vi "mediaBalls_v2.vi"(10 "Lado":enum16{"Esquerdo", "Direito"}(ring) caption="Enum", 11 "Array Ball Pose + CamID":T1(array[cluster])) -> (3 "Ball out":cluster{"x":dbl, "y":dbl})   [LabVIEW 2018]
panel:
  in  "cluster":cluster{"x":dbl, "y":dbl}
  in  "Field Size 2":T2
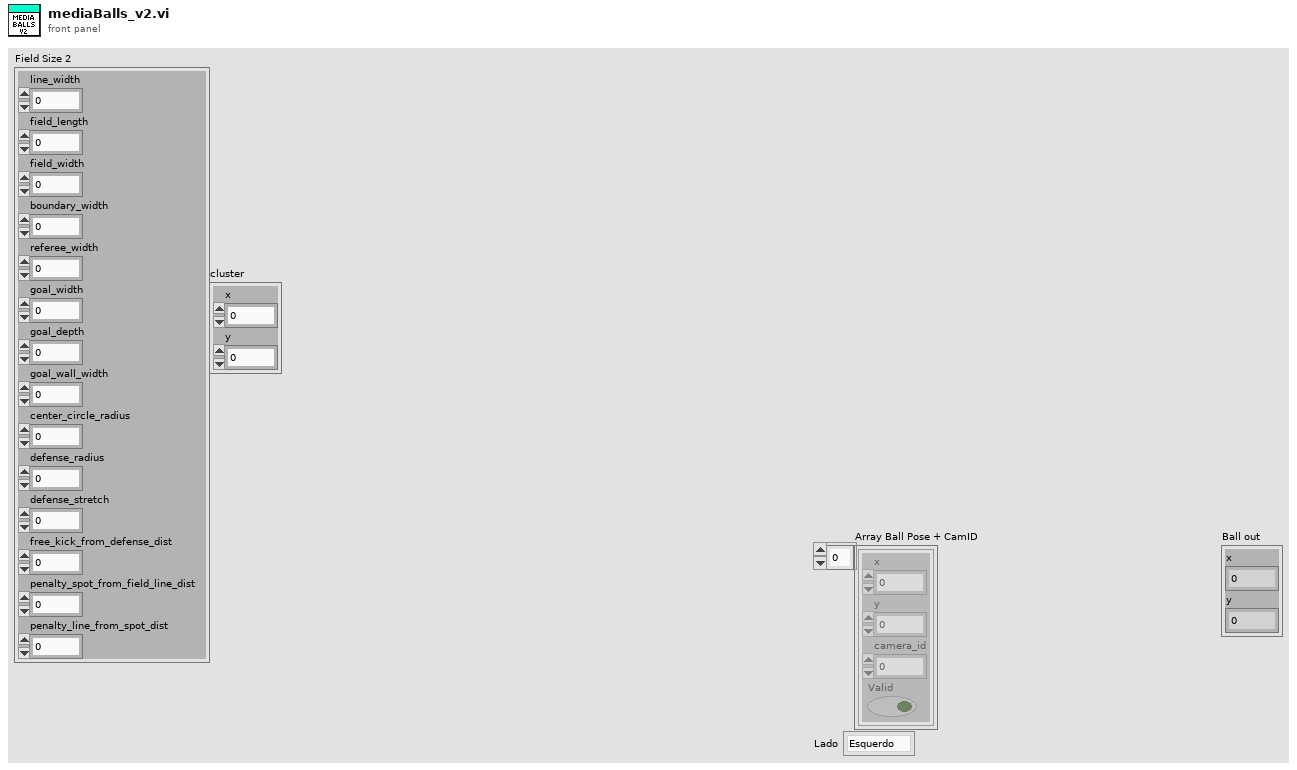
[diagram p1: front panel]
types:
  T1 = cluster{"x":sgl, "y":sgl, "camera_id":u32, "Valid":bool}[]
  T2 = cluster{"line_width":u32, "field_length":u32, "field_width":u32, "boundary_width":u32, "referee_width":u32, "goal_width":u32, "goal_depth":u32, "goal_wall_width":u32, "center_circle_radius":u32, "defense_radius":u32, "defense_stretch":u32, "free_kick_from_defense_dist":u32, "penalty_spot_from_field_line_dist":u32, "penalty_line_from_spot_dist":u32}
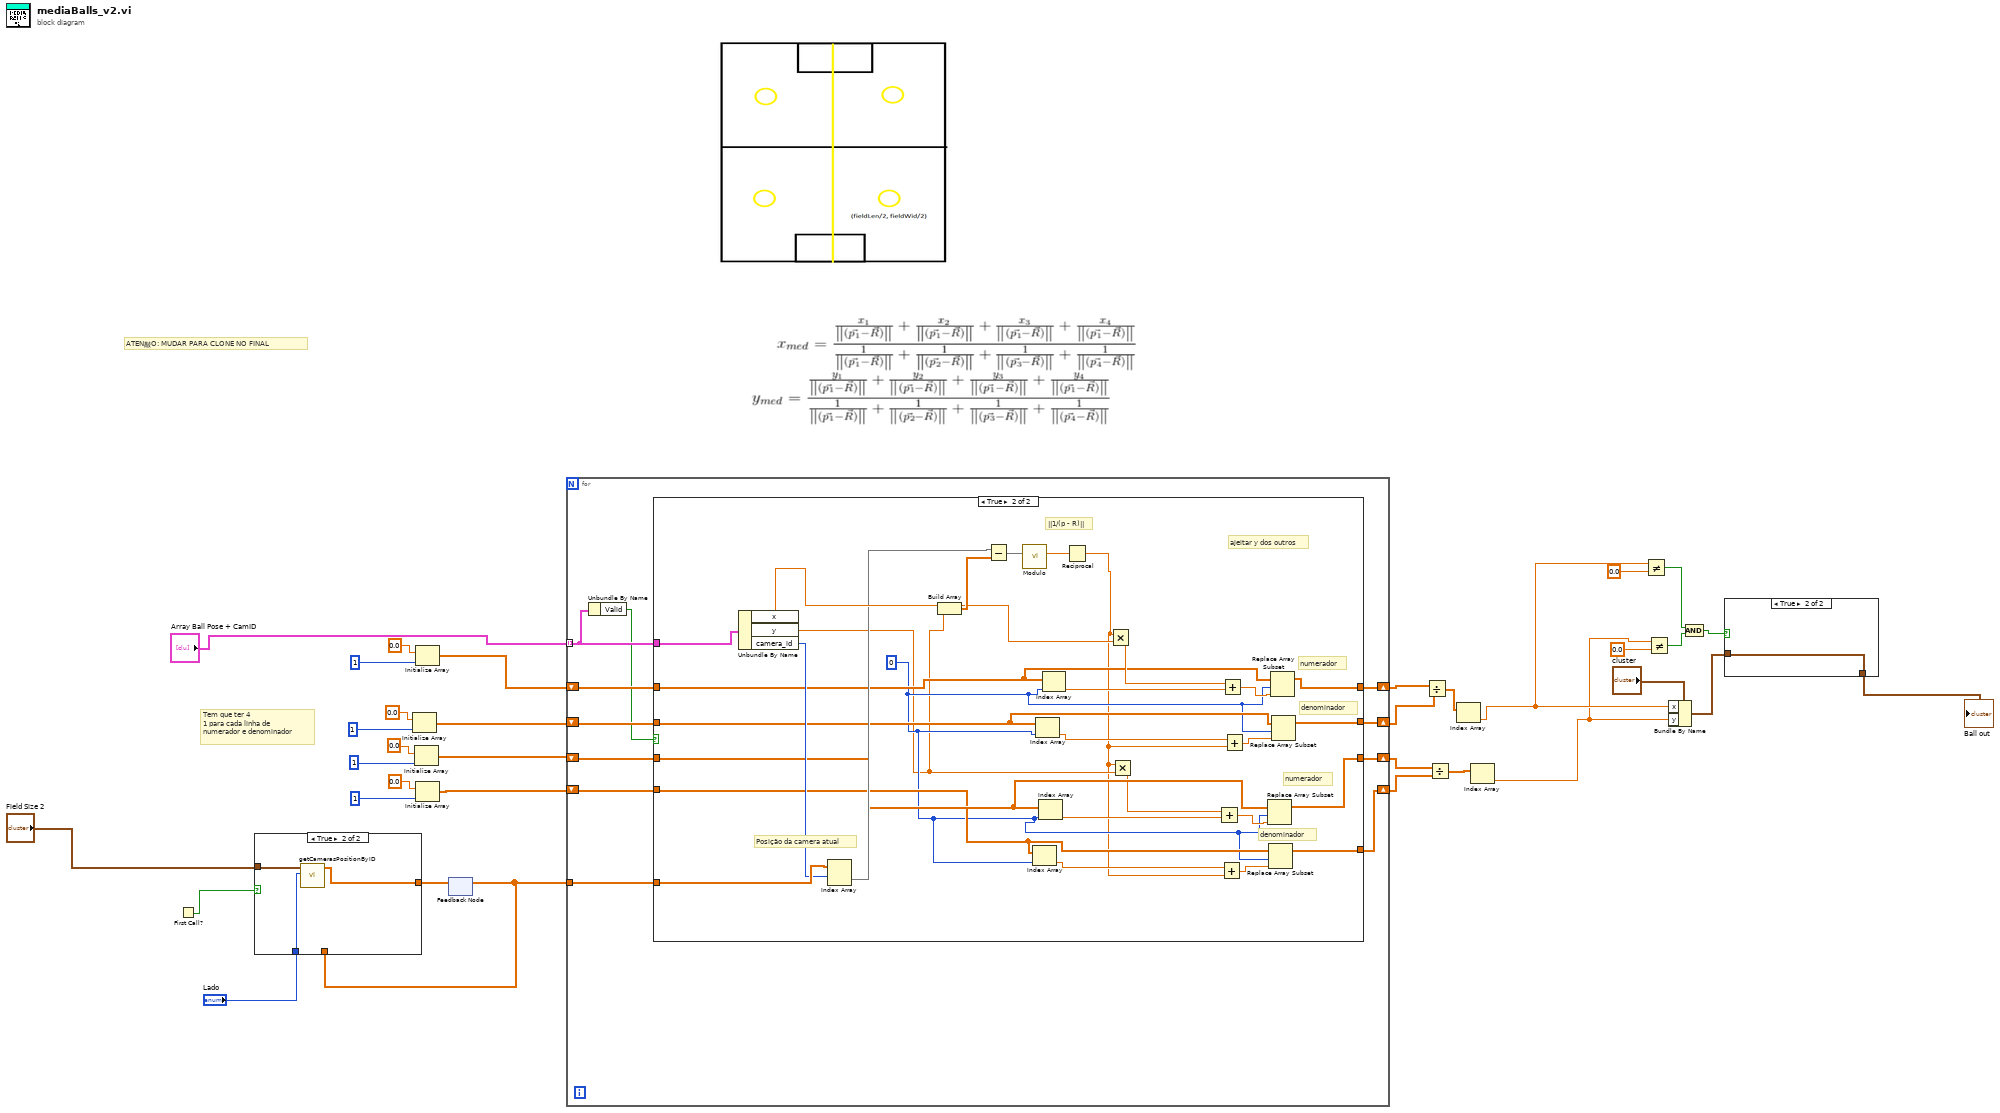
[diagram p0: block diagram]
diagram:
  # "Tem que ter 4\n1 para cada linha de\nnumerador e denominador"
  # "ATEN敲O: MUDAR PARA CLONE NO FINAL"
  n1 = First Call?() -> (First Call?: T/F=w4:bool)
  n2 = Initialize Array(0.0 ("element"), 1 ("dimension size")) -> (w25:dbl[])
  n3 = Initialize Array(0.0 ("element"), 1 ("dimension size")) -> (w24:dbl[])
  n4 = Initialize Array(0.0 ("element"), 1 ("dimension size")) -> (w26:dbl[])
  n5 = Initialize Array(0.0 ("element"), 1 ("dimension size")) -> (w23:dbl[])
  n6 = feedback #1() -> (w2:dbl[][])  [unwired: 1 in]
  n7 = case shown="True" w4 {
    tunnel: "Field Size 2" -> [_ w38]
    tunnel: [w35 w37] -> w3
    tunnel: w2 -> [w35 _]
    tunnel: "Lado" -> [_ w36]
    frame False {
    }
    frame True {
      n8 = call "getCamerasPositionByID.vi"("Lado"=w36, "Field Size 2"=w38) -> ("Cameras Positions"=w37:dbl[][])  [unwired: 9 in]
    }
  }
  n9 = feedback-in #1(w3) -> ()
  n10 = for {
    tunnel: "Array Ball Pose + CamID" -> [w40] mode=indexing
    tunnel: w2 -> [w49]
    shift-right: [w48] -> w22
    shift-left: w26 -> [w42]
    shift-right: [w47] -> w21
    shift-left: w25 -> [w41]
    shift-right: [w46] -> w20
    shift-left: w24 -> [w44]
    shift-right: [w45] -> w19
    shift-left: w23 -> [w43]
    n11 = Unbundle By Name(w40) -> ("Valid"=w39:bool)
    n12 = case shown="True" w39 {
      tunnel: w49 -> [_ w82]
      tunnel: [w53 w66] -> w48
      tunnel: [w52 w65] -> w47
      tunnel: [w51 w64] -> w46
      tunnel: [w50 w63] -> w45
      tunnel: w44 -> [w51 w62]
      tunnel: w43 -> [w50 w61]
      tunnel: w42 -> [w53 w60]
      tunnel: w41 -> [w52 w59]
      tunnel: w40 -> [_ w55]
      frame False {
      }
      frame True {
        w58 = 0 ("index")
        # "ajeitar y dos outros"
        # "denominador"
        # "numerador"
        # "denominador"
        # "numerador"
        # "||1/(p - R)||"
        # "Posição da camera atual"
        n13 = Unbundle By Name(w55) -> ("x"=w72:sgl, "y"=w57:sgl, "camera_id"=w81:u32)
        n14 = Index Array(array=w82, index (row)=w81) -> (element=w71:dbl[])  [unwired: 1 in]
        n15 = Build Array(w72, w57) -> (w80:sgl[])
        n16 = Subtract(x=w71, y=w80) -> (x-y=w79:dbl[])
        n17 = call "Modulo.vi"("2D vector"=w79) -> ("Modulo"=w78:dbl)  [unwired: 10 in]
        n18 = Index Array(array=w61, index=w58) -> (element=w67:dbl)
        n19 = Index Array(array=w59, index=w58) -> (element=w69:dbl)
        n20 = Index Array(array=w62, index=w58) -> (element=w68:dbl)
        n21 = Index Array(array=w60, index=w58) -> (element=w70:dbl)
        n22 = Reciprocal(x=w78) -> (1/x=w54:dbl)
        n23 = Multiply(x=w54, y=w72) -> (x*y=w77:dbl)
        n24 = Multiply(x=w54, y=w57) -> (x*y=w56:dbl)
        n25 = Add(x=w56, y=w68) -> (x+y=w74:dbl)
        n26 = Add(x=w67, y=w54) -> (x+y=w73:dbl)
        n27 = Add(x=w77, y=w70) -> (x+y=w76:dbl)
        n28 = Add(x=w69, y=w54) -> (x+y=w75:dbl)
        n29 = Replace Array Subset(array=w62, new element=w74, index=w58) -> (w64:dbl[])
        n30 = Replace Array Subset(array=w61, new element=w73, index=w58) -> (w63:dbl[])
        n31 = Replace Array Subset(array=w60, new element=w76, index=w58) -> (w66:dbl[])
        n32 = Replace Array Subset(array=w59, new element=w75, index=w58) -> (w65:dbl[])
      }
    }
  }
  n33 = Divide(x=w22, y=w21) -> (x/y=w11:dbl[])
  n34 = Divide(x=w20, y=w19) -> (x/y=w9:dbl[])
  n35 = Index Array(array=w11) -> (element=w10:dbl)  [unwired: 1 in]
  n36 = Index Array(array=w9) -> (element=w8:dbl)  [unwired: 1 in]
  n37 = Not Equal?(x=w10, y=0.0) -> (x != y?=w16:bool)
  n38 = Not Equal?(x=w8, y=0.0) -> (x != y?=w15:bool)
  n39 = Bundle By Name(cluster="cluster", "x"=w10, "y"=w8) -> (w13:cluster{"x":dbl, "y":dbl})
  n40 = And(x=w16, y=w15) -> (x .and. y?=w14:bool)
  n41 = case shown="True" w14 {
    tunnel: [w83 w84] -> w7
    tunnel: w13 -> [w83 w84]
    frame False {
    }
    frame True {
    }
  }
  "Ball out" <- w7
